vi "karel_read_osc_And.vi"(10 "file path":path=path "78-2009_11_26-12_33_00.dat") -> (0 "Шаг по времени, с":dbl, 1 "Количество точек":i32, 2 "Ch 1":waveform(i16), 3 "Ch 0":waveform(i16), 4 "Phase":dbl, 5 "Phase_Ok":bool, 6 "error out":errorcluster, 7 "t0":timestamp)   [LabVIEW 2010]
panel:
  out "Waveform Graph":waveform(i16)[](graph)
  # "Чтение осцилограммы из файла"
  # "Время московское (то, что настроено на измерителе)"
  # "Время местное"
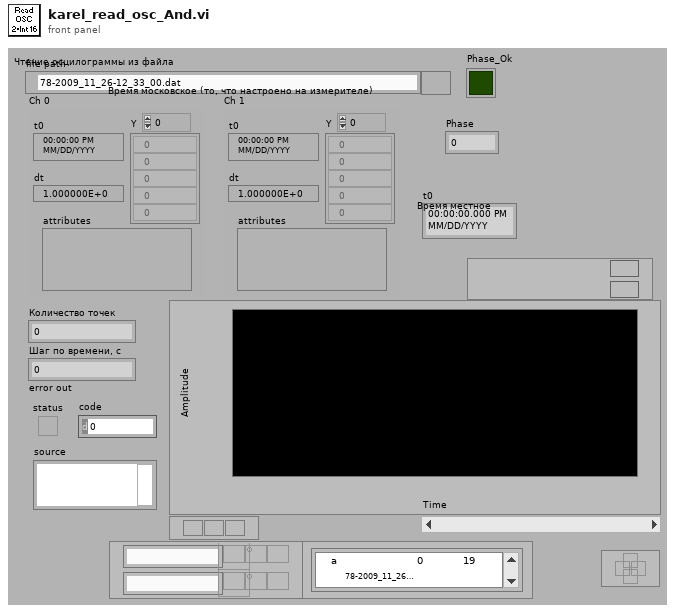
[diagram p1: front panel]
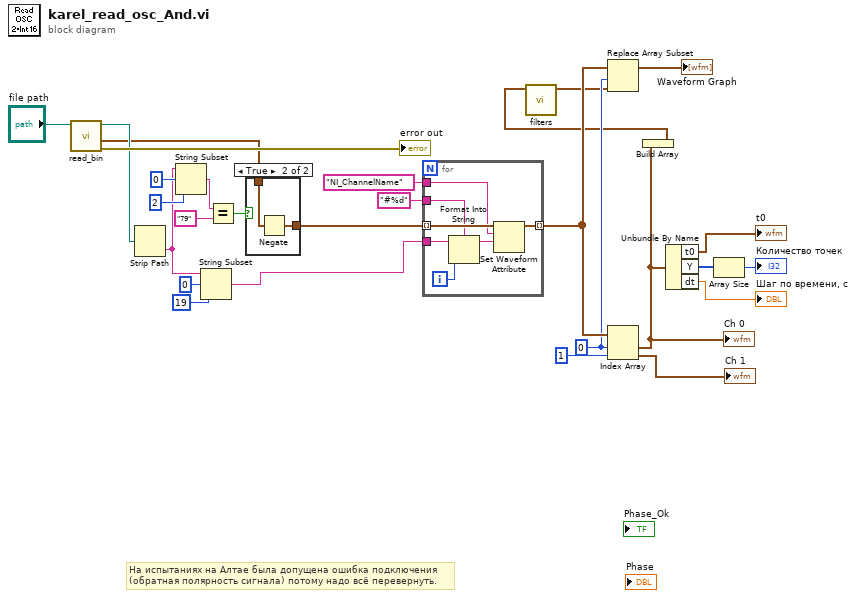
[diagram p0: block diagram]
diagram:
  w4 = 0 ("index")
  # "На испытаниях на Алтае была допущена ошибка подключения\n(обратная полярность сигнала) потому надо всё перевернуть."
  n1 = call "read_bin.vi"("datalog path"="file path") -> ("error out"=→"error out":errorcluster, "Waveform Graph"=w15:waveform(i16)[], "new file path"=w17:path)  [unwired: 3 in, 1 out]
  n2 = Strip Path(path=w17) -> (name=w23:string)  [unwired: 1 out]
  n3 = String Subset(string=w23, offset (0)=0, length (rest)=2 ("length (rest)")) -> (substring=w22:string)
  n4 = String Subset(string=w23, offset (0)=0, length (rest)=19 ("length (rest)")) -> (substring=w16:string)
  n5 = Equal?(x=w22, y="79") -> (x = y?=w20:bool)
  n6 = case shown="True" w20 {
    tunnel: w15 -> [w29 w31]
    tunnel: [w29 w30] -> w13
    frame False {
    }
    frame True {
      n7 = Negate(x=w31) -> (-x=w30:waveform(i16)[])
    }
  }
  n8 = for {
    tunnel: w16 -> [w37]
    tunnel: w13 -> [w35] mode=indexing
    tunnel: "NI_ChannelName" ("name") -> [w34]
    tunnel: "#%d" ("format string") -> [w33]
    tunnel: [w32] -> w6 mode=indexing
    i -> [w38]
    n9 = Format Into String(format string=w33, initial string=w37, w38) -> (resulting string=w36:string)  [unwired: 1 in, 1 out]
    n10 = Set Waveform Attribute(5:w36, 6:w34, 7:w35) -> (3:w32:waveform(i16))  [unwired: 1 in, 2 out]
  }
  n11 = Index Array(array=w6, index #1=w4, index #2=1 ("index")) -> (element #1=w3:waveform(i16), element #2=→"Ch 1":waveform(i16))
  "Ch 0" <- w3
  n12 = Build Array(w3) -> (w2:waveform(i16)[])
  n13 = call "filters.vi"("Array"=w2) -> ("Array 2"=w1:waveform(i16)[])  [unwired: 6 in]
  n14 = Replace Array Subset(array=w6, new element=w1, index=w4) -> (→"Waveform Graph":waveform(i16)[])
  n15 = Unbundle By Name(w3) -> ("t0"=→"t0":timestamp, "Y"=w9:i16[], "dt"=→"Шаг по времени, с":dbl)
  n16 = Array Size(array=w9) -> (size(s)=→"Количество точек":i32)
